vi "ctx set max sample delay seconds.vi"(10 "max_data_delay_seconds":u16, 11 "context":u32) -> (2 "function return":i32, 3 "context out":u32)   [LabVIEW 2019, in "apdm.lvlib"]
doc: "APDM_EXPORT int apdm_ctx_set_max_sample_delay_seconds(apdm_ctx_t context, const uint16_t max_data_delay_seconds);"
uses:
  apdm.lvlib
  Lee Lab/CP FES Walking 2018/Code/Working/LabVIEW/apdm.dll
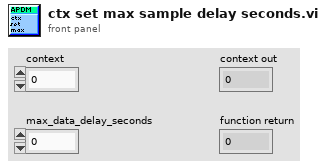
[diagram p1: front panel]
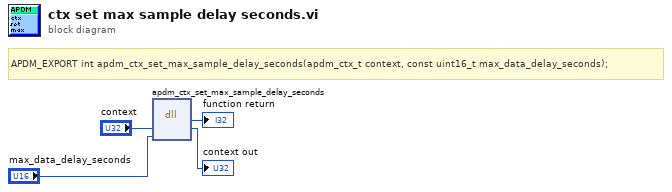
[diagram p0: block diagram]
diagram:
  # "APDM_EXPORT int apdm_ctx_set_max_sample_delay_seconds(apdm_ctx_t context, const uint16_t max_data_delay_seconds);"
  n1 = dll-call lib="C:/Users/jfalesi/Dropbox/Lee Lab/CP FES Walking 2018/Code/Working/LabVIEW/apdm.*" fn="apdm_ctx_set_max_sample_delay_seconds"("context"="context", "max_data_delay_seconds"="max_data_delay_seconds") -> (→"function return":i32, "context"=→"context out":u32)  [unwired: 4 in, 2 out]
